vi "lfieldpanel_DO_connect.vi"(8 "error in (no error)":errorcluster, 10 "Is Visible?":bool=TRUE, 11 "lightfield_panel in":refnum<class "lightfield_panel.lvclass">) -> (0 "error out":errorcluster, 3 "lightfield_panel out":refnum<class "lightfield_panel.lvclass">)   [LabVIEW 2015, in "lightfield_panel.lvclass"]
uses:
  lightfield_panel.lvclass
  lightfield/lightfield_class.lvclass
  lightfield_panel.lvclass/lightfield_panel.ctl
  lightfield/lightfield_class.lvclass/lightfield_class.ctl
  UI/panel_class/panel.lvclass
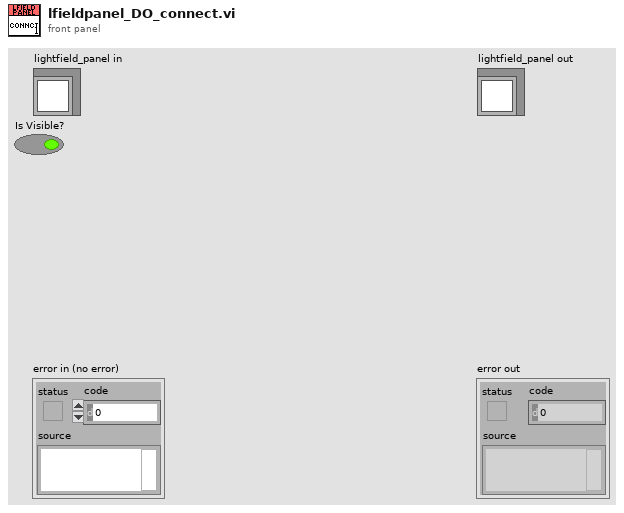
[diagram p1: front panel]
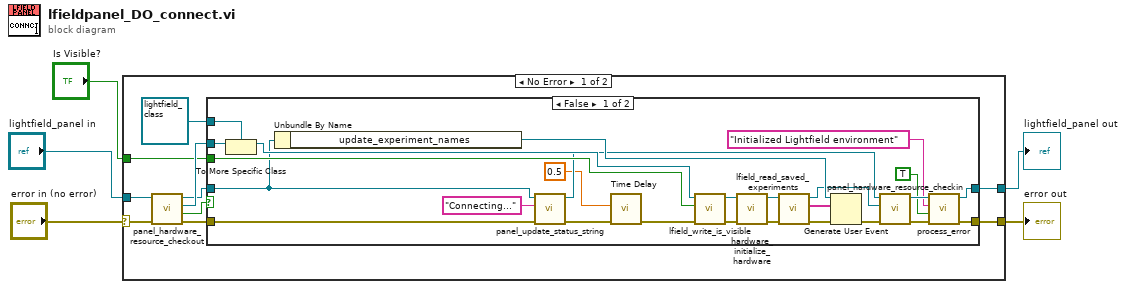
[diagram p0: block diagram]
diagram:
  n1 = case shown="No Error" "error in (no error)" {
    selector: "error in (no error)" -> [w14 w45]
    tunnel: [w8 w45] -> w4
    tunnel: [w7 w44] -> w2
    tunnel: "lightfield_panel in" -> [w15 w44]
    tunnel: "Is Visible?" -> [w6 _]
    frame No Error {
      n2 = call "panel_hardware_resource_checkout.vi"("error in (no error)"=w14, "panel in"=w15) -> ("error out"=w10:errorcluster, "timed out?"=w13:bool, "hardware.lvclass"=w11:refnum<class "hardware.lvclass">, "panel out"=w9:refnum<class "lightfield_panel.lvclass">)  [unwired: 6 in]
      n3 = case shown="False" w13 {
        tunnel: refnum<class "lightfield_class.lvclass"> refnum ("lightfield_class.lvclass") -> [w41 _]
        tunnel: w11 -> [w40 _]
        tunnel: w10 -> [w22 w42]
        tunnel: w9 -> [w21 w43]
        tunnel: [w30 w42] -> w8
        tunnel: [w29 w43] -> w7
        tunnel: w6 -> [w25 _]
        frame False {
          n4 = To More Specific Class(target class=w41, reference=w40) -> (specific class reference=w27:refnum<class "lightfield_class.lvclass">)  [unwired: 1 in, 1 out]
          n5 = Unbundle By Name(w21) -> ("update_experiment_names"=w37:refnum<user-event>)
          n6 = call-dynamic "panel_update_status_string.vi"("error in (no error)"=w22, "String"="Connecting...", "lightfield_panel in"=w21) -> ("error out"=w18:errorcluster, "lightfield_panel out"=w20:refnum<class "lightfield_panel.lvclass">)  [unwired: 7 in]
          n7 = call "Time Delay"("error in (no error)"=w18, "Delay Time (s)"=0.5) -> ("error out"=w17:errorcluster)  [unwired: 9 in]
          n8 = call "lfield_write_is_visible.vi"("error in (no error)"=w17, "Is Visible?"=w25, "lightfield_class in"=w27) -> ("error out"=w28:errorcluster, "lightfield_class out"=w26:refnum<class "lightfield_class.lvclass">)  [unwired: 7 in]
          n9 = call-dynamic "hardware_initialize_hardware.vi"("error in (no error)"=w28, "lightfield_class in"=w26) -> ("error out"=w39:errorcluster, "lightfield_class out"=w38:refnum<class "lightfield_class.lvclass">)  [unwired: 8 in]
          n10 = call-dynamic "lfield_read_saved_experiments.vi"("error in (no error)"=w39, "lightfield_class in"=w38) -> ("error out"=w33:errorcluster, "Saved Experiments"=w36:string[], "lightfield_class out"=w35:refnum<class "lightfield_class.lvclass">)  [unwired: 7 in]
          n11 = Generate User Event(user event=w37, event data cluster=w36, error in=w33) -> (error out=w31:errorcluster)  [unwired: 1 in, 1 out]
          n12 = call "panel_hardware_resource_checkin.vi"("error in (no error)"=w31, "hardware.lvclass"=w35, "panel in"=w20) -> ("error out"=w32:errorcluster, "panel out"=w34:refnum<class "lightfield_panel.lvclass">)  [unwired: 7 in]
          n13 = call "process_error.vi"("error in (no error)"=w32, "Update Status"=TRUE, "No Error Message"="Initialized Lightfield environment", "lightfield_panel in"=w34) -> ("error out"=w30:errorcluster, "lightfield_panel out"=w29:refnum<class "lightfield_panel.lvclass">)  [unwired: 6 in]
        }
        frame True {
        }
      }
    }
    frame Error {
    }
  }
  "error out" <- w4
  "lightfield_panel out" <- w2
